vi "Get LeftKey.vi"(8 "error in (no error)":errorcluster, 11 "senseHatJoystick in":refnum<class "RPI.SenseHat.Joystick.lvclass">) -> (0 "error out":errorcluster, 3 "senseHatJoystick out":refnum<class "RPI.SenseHat.Joystick.lvclass">)   [LabVIEW 2020, in "RPI.SenseHat.Joystick.lvlib" / "RPI.SenseHat.Joystick.lvclass"]
uses:
  RPI.SenseHat.Joystick.lvclass
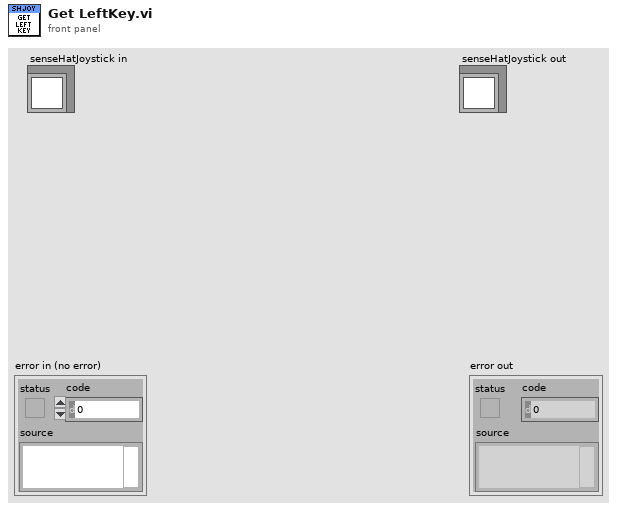
[diagram p1: front panel]
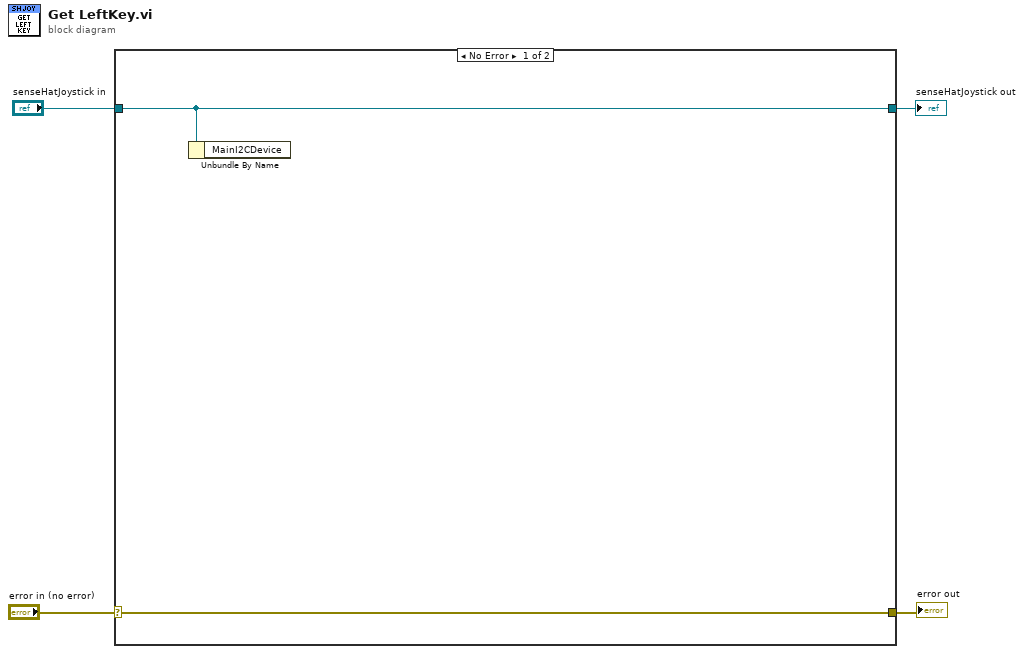
[diagram p0: block diagram]
diagram:
  n1 = case shown="No Error" "error in (no error)" {
    selector: "error in (no error)" -> [w6 w8]
    tunnel: [w6 w8] -> w3
    tunnel: [w5 w7] -> w1
    tunnel: "senseHatJoystick in" -> [w5 w7]
    frame No Error {
      n2 = Unbundle By Name(w5) -> ()  [unwired: 1 out]
    }
    frame Error {
    }
  }
  "error out" <- w3
  "senseHatJoystick out" <- w1
